vi "MecaKinematics_ToTwist2d.vi"(9 "Wheel Deltat Positions":T4 {"RearRight" format="%19.3f"; "RearLeft" format="%19.3f"; "FrontRight" format="%19.3f"; "FrontLeft" format="%19.3f"}, 11 "in MECA_DRIVE_KINEMATICS":T1={"FrontLeft"={"X"=0.0, "Y"=0.0}, "FrontRight"={"X"=0.0, "Y"=0.0}, "RearLeft"={"X"=0.0, "Y"=0.0}, "RearRight"={"X"=0.0, "Y"=0.0}, "InverseKinematics"=[[0.0, 1.0, -1.0, 0.0], [0.0, 1.0, 1.0, 0.0], [0.0, 1.0, 1.0, 0.0], [0.0, 1.0, -1.0, 0.0]], "ForwardKinematics"=[[0.0, 1.0, -1.0, 0.0], [0.0, 1.0, 1.0, 0.0], [0.0, 1.0, 1.0, 0.0], [0.0, 1.0, -1.0, 0.0]], "PrevCoR"={"X"=0.0, "Y"=0.0}} {"PrevCoR"."Y" format="%14.3f"; "PrevCoR"."X" format="%14.3f"; "RearRight"."Y" format="%14.3f"; "RearRight"."X" format="%14.3f"; "RearLeft"."Y" format="%14.3f"; "RearLeft"."X" format="%14.3f"; "FrontRight"."Y" format="%14.3f"; "FrontRight"."X" format="%14.3f"; "FrontLeft"."Y" format="%14.3f"; "FrontLeft"."X" format="%14.3f"}) -> (3 "Twist2d":T5)   [LabVIEW 2019, in "Trajectory_Library.lvlib"]
doc: "Performs forward kinematics to return the resulting Twist2d from the given wheel deltas. This method is often used for odometry -- determining the robot's position on the field using changes in the distance driven by each wheel on the robot.\n \n * @param \n * @return The resulting Twist2d.\n\nParametetrs:\n - MecaDriveKinematics -- Data structure\n - wheelDeltas -- The distances driven by each wheel.\n\nReturns:\n - Twist2d - The resulting twist."
uses:
  Trajectory_Library.lvlib
  TypeDef/TWIST2D.ctl
  TypeDef/MECA_WHEEL_POSITIONS.ctl
  TypeDef/MECA_DRIVE_KINEMATICS.ctl
  TypeDef/TRANSLATION2D.ctl
  <vilib>/Analysis/Matrix/Datatypes/RealMatrix.ctl
  MatrixHelper_CoerceSize.vi
  <vilib>/Analysis/Matrix/Numeric/Multiply/Multiply - RM,RM.vi
  <vilib>/Analysis/Matrix/NI_Matrix.lvlib
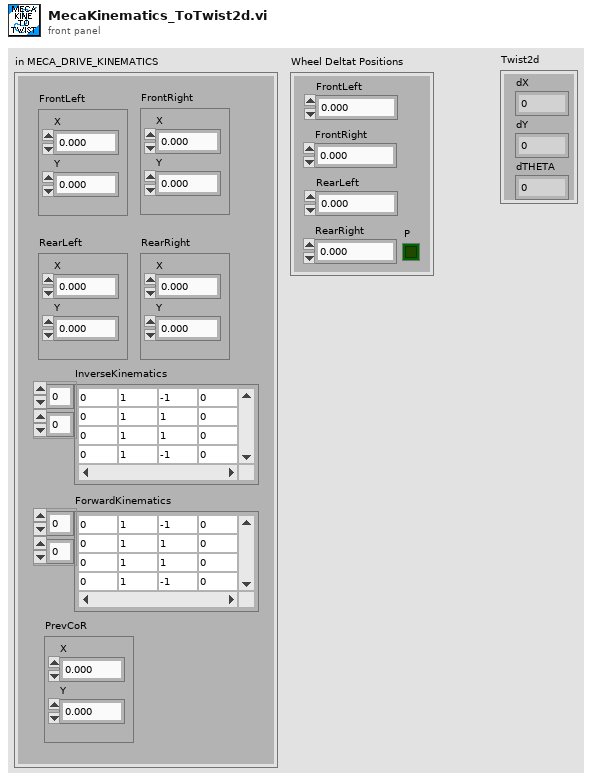
[diagram p1: front panel]
types:
  T1 = typedef "Trajectory_Library.lvlib/MECA_DRIVE_KINEMATICS.ctl" = cluster{"FrontLeft":T2, "FrontRight":T2, "RearLeft":T2, "RearRight":T2, "InverseKinematics":T3, "ForwardKinematics":T3, "PrevCoR":T2}
  T2 = typedef "Trajectory_Library.lvlib/TRANSLATION2D.ctl" = cluster{"X":dbl, "Y":dbl}
  T3 = typedef "NI_Matrix.lvlib/RealMatrix.ctl" = dbl[][]
  T4 = typedef "Trajectory_Library.lvlib/MECA_WHEEL_POSITIONS.ctl" = cluster{"FrontLeft":dbl, "FrontRight":dbl, "RearLeft":dbl, "RearRight":dbl, "P":bool}
  T5 = typedef "Trajectory_Library.lvlib/TWIST2D.ctl" = cluster{"dX":dbl, "dY":dbl, "dTHETA":dbl}
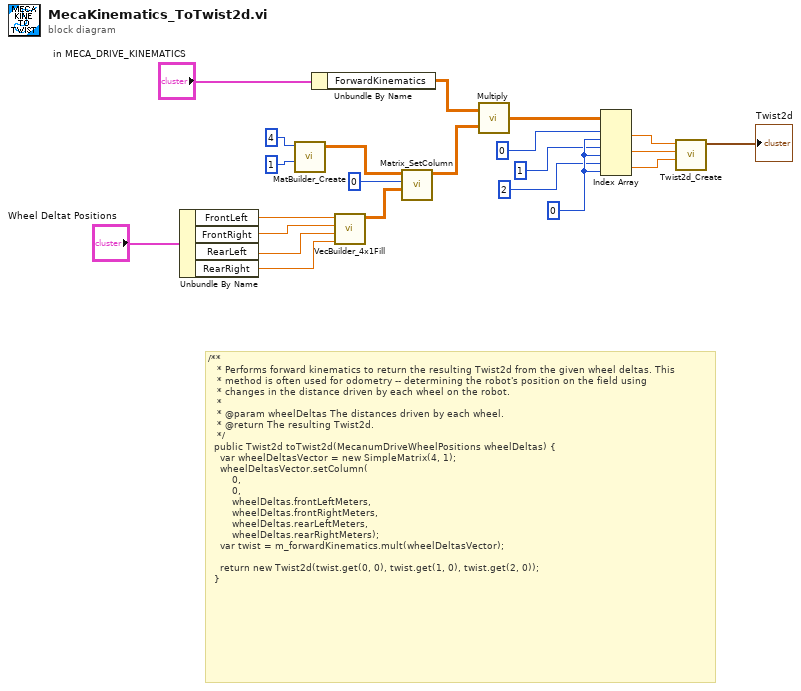
[diagram p0: block diagram]
diagram:
  w22 = 0 ("index (col)")
  # "/**\n   * Performs forward kinematics to return the resulting Twist2d from the given wheel deltas. This\n   * method is often used for odometry -- determining the robot's position on the field using\n   * changes in the distance driven by each wheel on the robot.\n   *\n   * @param wheelDeltas The distances driven by each wheel.\n   * @return The resulting Twist2d.\n   */\n  public Twist2d toTwist2d(MecanumDriveWheelPositions wheelDeltas) {\n    var wheelDeltasVector = new SimpleMatrix(4, 1);\n    wheelDeltasVector.setColumn(\n        0,\n        0,\n        wheelDeltas.frontLeftMeters,\n        wheelDeltas.frontRightMeters,\n        wheelDeltas.rearLeftMeters,\n        wheelDeltas.rearRightMeters);\n    var twist = m_forwardKinematics.mult(wheelDeltasVector);\n\n    return new Twist2d(twist.get(0, 0), twist.get(1, 0), twist.get(2, 0));\n  }"
  n1 = Unbundle By Name("Wheel Deltat Positions") -> ("FrontLeft"=w4:dbl, "FrontRight"=w3:dbl, "RearLeft"=w2:dbl, "RearRight"=w1:dbl)
  n2 = call "MatBuilder_Create.vi"("Columns"=1, "Rows"=4) -> ("output matrix"=w9:T3)  [unwired: 9 in]
  n3 = Unbundle By Name("in MECA_DRIVE_KINEMATICS") -> ("ForwardKinematics"=w17:T3)
  n4 = call "VecBuilder_4x1Fill.vi"("R3"=w1, "R2"=w2, "R1"=w3, "R0"=w4) -> ("output matrix"=w7:T3)  [unwired: 7 in]
  n5 = call "Matrix_SetColumn.vi"("Fill Vector"=w7, "Column"=0, "input matrix"=w9) -> ("output matrix"=w6:T3)  [unwired: 7 in, 1 out]
  n6 = call-poly <vilib>:"Multiply.vi"("Real Matrix B"=w6, "Real Matrix A"=w17) -> ("A * B"=w16:T3)
  n7 = Index Array(array=w16, index (row) #1=0 ("index (row)"), index (col) #1=w22, index (row) #2=1 ("index (row)"), index (col) #2=w22, index (row) #3=2 ("index (row)"), index (col) #3=w22) -> (element #1=w15:dbl, element #2=w14:dbl, element #3=w13:dbl)
  n8 = call "Twist2d_Create.vi"("dTHETA"=w13, "dY"=w14, "dX"=w15) -> ("TWIST"=→"Twist2d":T5)  [unwired: 8 in]
